vi "Elevator Controller.vi"(8 "error in":errorcluster) -> ()   [LabVIEW 2018]
doc: "This VI executes continuously carrying out the current operation and responding to updates or new operations. It will often contain the timing or control code that is difficult to place directly in TeleOp. This VI generally opens all sensors and motors and isolates the rest of the robot code from knowing how the operations are carried out."
uses:
  Elevator Setpoints.ctl
  Elevator Operations.ctl
  <vilib>/Rock Robotics/WPI/ThirdParty/Phoenix-LabVIEW/Motor Controller/Controls/CTRE_Phoenix_MotorControl_NeutralMode.ctl
  <vilib>/Rock Robotics/WPI/ThirdParty/Phoenix-LabVIEW/Motor Controller/Controls/CTRE_Phoenix_MotorControl_ControlMode.ctl
  <vilib>/Rock Robotics/WPI/ThirdParty/Phoenix-LabVIEW/Motor Controller/Controls/CTRE_Phoenix_MotorControl_FeedbackDevice.ctl
  <vilib>/Rock Robotics/SystemInterfaces/DIO/FPGA_DIOChannel.ctl
  <vilib>/Rock Robotics/WPI/ThirdParty/Phoenix-LabVIEW/Motor Controller/Get/CTRE_Phoenix_MotorController_GetQuadratureData.vi
  <vilib>/Rock Robotics/Network Tables/NT Write Number.vi
  <vilib>/Rock Robotics/Network Tables/NT Write Boolean.vi
panel:
  out "Current\nCmd":string
  # "Tip: It may be helpful to observe inputs and sensor values.\nYou may also want to display tuning or debugging controls."
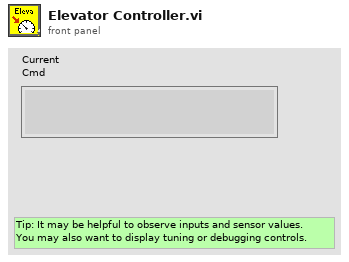
[diagram p1: front panel]
types:
  T1 = typedef "FPGA_DIOChannel.ctl" = enum8{"DIO 0", "DIO 1", "DIO 2", "DIO 3", "DIO 4", "DIO 5", "DIO 6", "DIO 7", "DIO 8", "DIO 9", "DIO MXP 0", "DIO MXP 1", "DIO MXP 2", "DIO MXP 3", "DIO MXP 4", "DIO MXP 5", "DIO MXP 6", "DIO MXP 7", "DIO MXP 8", "DIO MXP 9", "DIO MXP 10", "DIO MXP 11", "DIO MXP 12", "DIO MXP 13", "DIO MXP 14", "DIO MXP 15", "SPI Port CS1", "SPI Port CS2", "SPI Port CS3", "SPI Port MISO", "SPI Port MOSI", "Invalid"}
  T2 = typedef "CTRE_Phoenix_MotorControl_FeedbackDevice.ctl" = i8
  T3 = typedef "CTRE_Phoenix_MotorControl_ControlMode.ctl" = u16
  T4 = typedef "CTRE_Phoenix_MotorControl_NeutralMode.ctl" = enum8{"EEPROMSetting", "Override to Coast", "Override to Brake"}
  T5 = typedef "Elevator Setpoints.ctl" = cluster{"Operation":T6, "Setpoint":dbl, "Duration":dbl}
  T6 = typedef "Elevator Operations.ctl" = enum16{"Reserve", "Read Current", "Immediate", "Move Elevator", "Elevator Preset", "Elevator For Time"}
  T7 = typedef "WPI_MotorControlDeviceRef.ctl" = cluster{"DeviceStatus":errorcluster, "Type":T8, "PWM":cluster{"PWM Channel":T9, "DeadBand":T10}, "CAN":cluster{"Device Number":u8, "SetOutput VI Ref":variant, "GetOutput VI Ref":variant, "Enable VI Ref":variant, "Disable VI Ref":variant, "Data":variant}, "Invert":bool, "DIO PWM":cluster{"PWM \"Enable\" Channel":T9, "DIOChannel":T1, "PWM Rate":dbl}}
  T8 = typedef "WPI_MotorControlType.ctl" = enum16{"PWM", "CAN", "DIO PWM"}
  T9 = typedef "FPGA_DIOPWMChannel.ctl" = enum8{"PWM 0", "PWM 1", "PWM 2", "PWM 3", "PWM 4", "PWM 5", "PWM 6", "PWM 7", "PWM 8", "PWM 9", "PWM MXP 0", "PWM MXP 1", "PWM MXP 2", "PWM MXP 3", "PWM MXP 4", "PWM MXP 5", "PWM MXP 6", "PWM MXP 7", "PWM MXP 8", "PWM MXP 9", "Invalid"}
  T10 = typedef "WPI_PWMDeadband.ctl" = cluster{"Name":string, "maxPositivePwm":i32, "minPositivePwm":i32, "centerPwm":i32, "maxNegativePwm":i32, "minNegativePwm":i32, "angularRange":u16}
  T11 = typedef "Command Status Info.ctl" = cluster{"Name":string, "Status":T12, "notifier out":T13}
  T12 = typedef "Completion Status.ctl" = enum16{"Successful", "Aborted", "Incomplete"}
  T13 = typedef "Completion Notifier.ctl" = refnum<notifier>
  T14 = cluster{"Current Command":T5, "Command Timing":cluster{"Start Time (ms)":u32, "Iterations":i32}, "Command Arguments":cluster{"Command Info":T11, "Description":string, "Default Command":T5, "queue out":refnum<queue>, "Subsystem Name":string}}
  T15 = typedef "WPI_DigitalInputDevRef.ctl" = cluster{"DevStatus":errorcluster, "DIO Channel":T1}
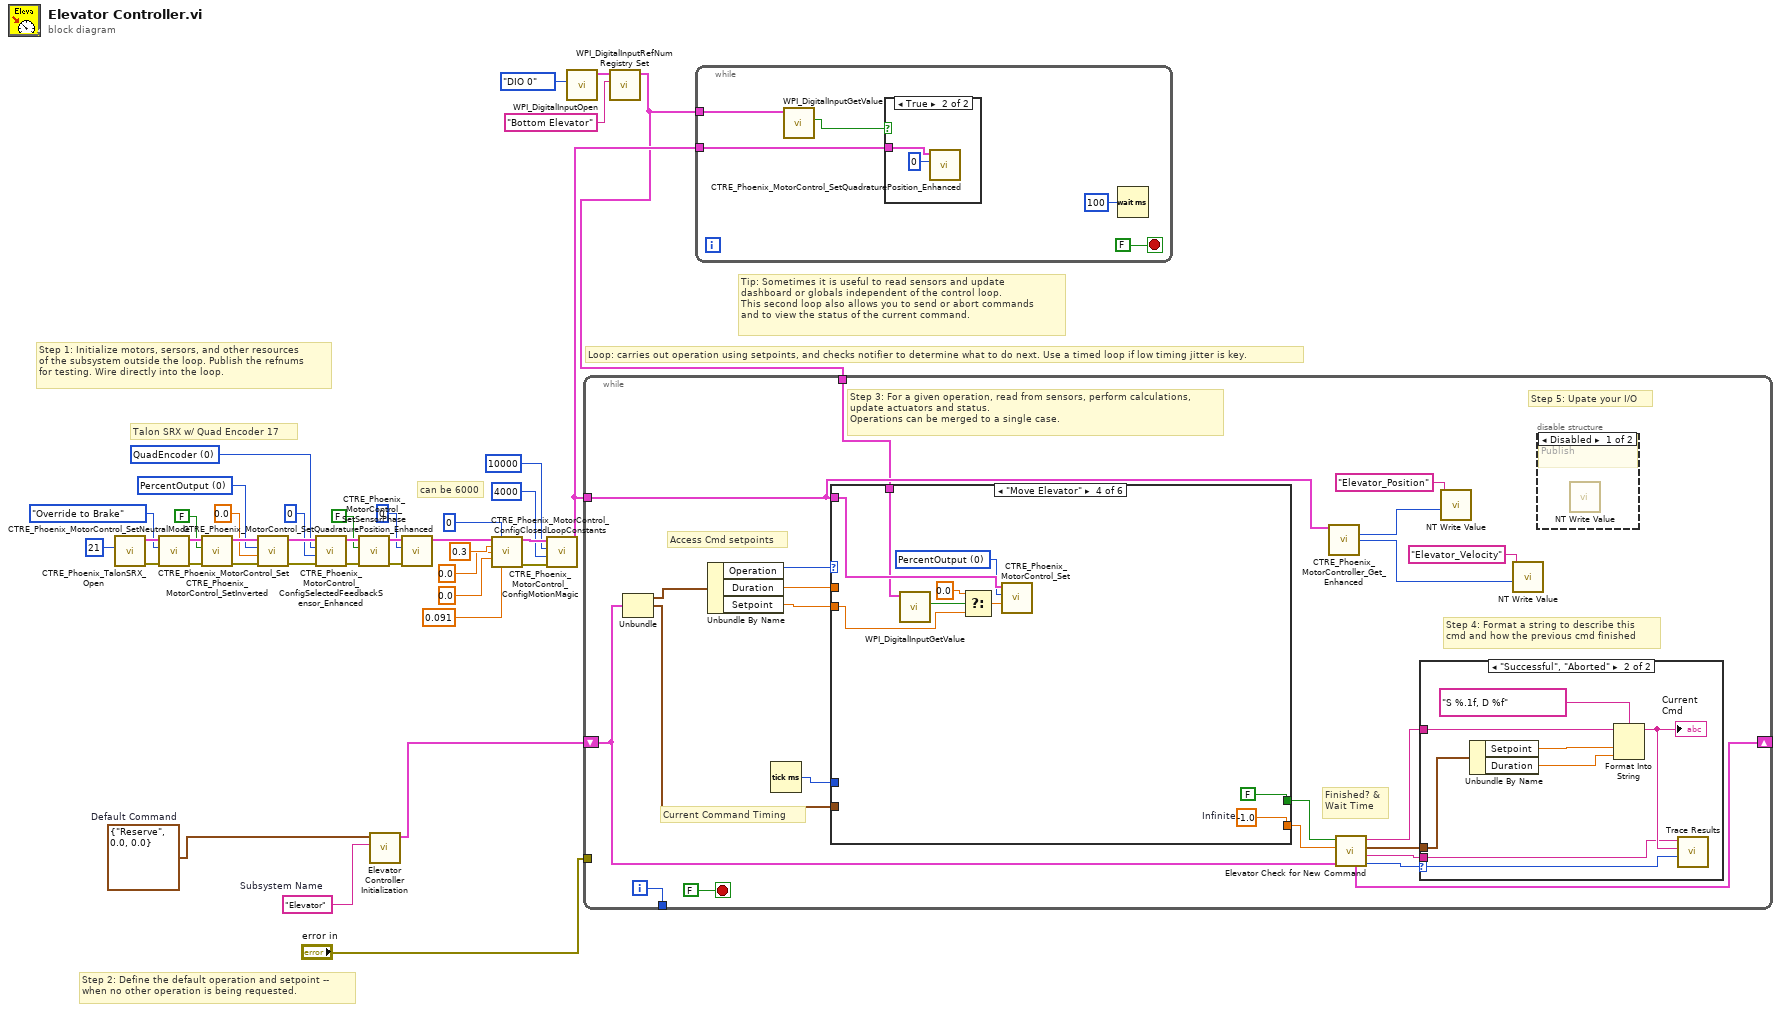
[diagram p0: block diagram]
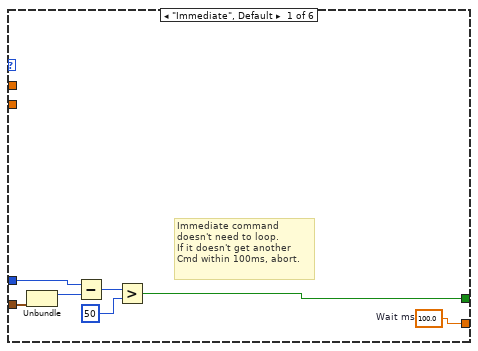
[diagram p5: hidden frame]
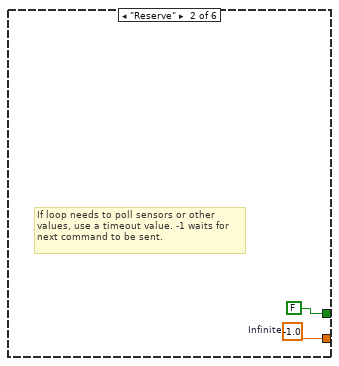
[diagram p6: hidden frame]
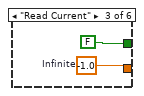
[diagram p7: hidden frame]
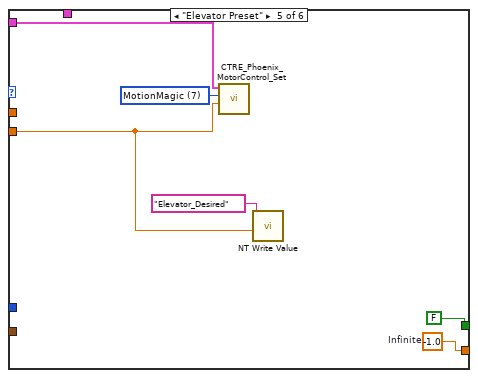
[diagram p8: hidden frame]
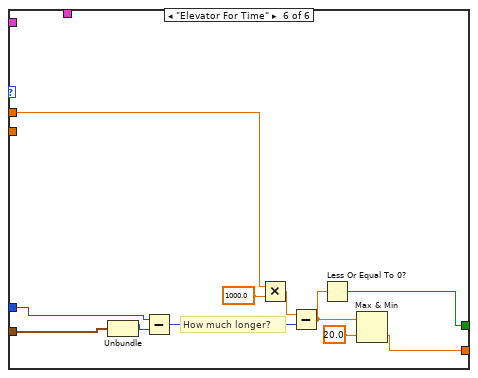
[diagram p9: hidden frame]
diagram:
  w19 = T2 0 items=["QuadEncoder"=0, "Analog"=2, "Tachometer"=4, "Pulse Width Encoded Position"=8, "Sensor Sum (S0 + S1)"=9, "Sensor Difference (D0 - D1)"=10, "Remote Source 0"=11, "Remote Source 1"=12, "Software Emulated"=15] ("Feedback Device")
  w21 = T3 0 items=["PercentOutput"=0, "Position"=1, "Velocity"=2, "Current"=3, "Follower"=5, "MotionProfile"=6, "MotionMagic"=7, "MotionProfileArc"=10, "Disabled"=15] ("Control Mode")
  w37 = T5 {"Operation"=enum."Reserve", "Setpoint"=0.0, "Duration"=0.0}  # Default Command
  w38 = "Elevator"  # Subsystem Name
  # "can be 6000"
  # "Talon SRX w/ Quad Encoder 17"
  # "Tip: Sometimes it is useful to read sensors and update\ndashboard or globals independent of the control loop.\nThis second loop also allows you to send or abort commands\nand to view the status of the current command."
  # "Step 2: Define the default operation and setpoint --\nwhen no other operation is being requested."
  # "Step 1: Initialize motors, sersors, and other resources\nof the subsystem outside the loop. Publish the refnums\nfor testing. Wire directly into the loop."
  # "Loop: carries out operation using setpoints, and checks notifier to determine what to do next. Use a timed loop if low timing jitter is key."
  n1 = call <vilib>:"CTRE_Phoenix_TalonSRX_Open.vi"("Device Number"=u8 21) -> ("error out"=w26:errorcluster, "CAN Talon SRX Ref"=w25:T7)  [unwired: 9 in]
  n2 = call <vilib>:"CTRE_Phoenix_MotorControl_SetNeutralMode.vi"("error in (no error)"=w26, "Motor Control Neutral Mode"=CTRE_Phoenix_MotorControl_NeutralMode."Override to Brake", "PhoenixMotorControlDevRef"=w25) -> ("error out"=w36:errorcluster, "PhoenixMotorControlDevRef"=w35:T7)  [unwired: 7 in]
  n3 = call <vilib>:"CTRE_Phoenix_MotorControl_SetInverted.vi"("error in (no error)"=w36, "Invert?"=FALSE, "PhoenixMotorControlDevRef"=w35) -> ("error out"=w34:errorcluster, "PhoenixMotorControlDevRef"=w33:T7)  [unwired: 7 in]
  n4 = call <vilib>:"CTRE_Phoenix_MotorControl_Set.vi"("error in (no error)"=w34, "Output"=0.0, "Control Mode"=w21, "PhoenixMotorControlDevRef"=w33) -> ("error out"=w27:errorcluster, "PhoenixMotorControlDevRef"=w32:T7)  [unwired: 6 in]
  n5 = call <vilib>:"CTRE_Phoenix_MotorControl_ConfigSelectedFeedbackSensor_Enhanced.vi"("error in (no error)"=w27, "pidLoopIdx"=0, "Feedback Device"=w19, "PhoenixMotorControlDevRef"=w32) -> ("error out"=w28:errorcluster, "PhoenixMotorControlDevRef"=w31:T7)  [unwired: 6 in]
  n6 = call <vilib>:"CTRE_Phoenix_MotorControl_SetSensorPhase.vi"("error in (no error)"=w28, "PhaseSensor"=FALSE, "PhoenixMotorControlDevRef"=w31) -> ("error out"=w29:errorcluster, "PhoenixMotorControlDevRef"=w30:T7)  [unwired: 7 in]
  n7 = call "Elevator Controller Initialization.vi"("Subsystem Name"=w38, "Default Command"=w37) -> ("Current Command"=w39:T14)  [unwired: 9 in]
  n8 = call <vilib>:"CTRE_Phoenix_MotorControl_SetQuadraturePosition_Enhanced.vi"("error in (no error)"=w29, "New Position"=0, "PhoenixMotorControlDevRef"=w30) -> ("PhoenixMotorControlDevRef"=w13:T7)  [unwired: 7 in, 1 out]
  n9 = call <vilib>:"CTRE_Phoenix_MotorControl_ConfigClosedLoopConstants.vi"("PhoenixMotorControlDevRef"=w13, "slotIdx"=0, "P"=0.3, "I"=0.0, "D"=0.0, "F"=0.091) -> ("PhoenixMotorControlDevRef"=w16:T7, "error out"=w17:errorcluster)  [unwired: 8 in]
  n10 = call <vilib>:"CTRE_Phoenix_MotorControl_ConfigMotionMagic.vi"("error in (no error)"=w17, "Acceleration"=4000, "Cruise Velocity"=10000, "PhoenixMotorControlDevRef"=w16) -> ("PhoenixMotorControlDevRef"=w5:T7)  [unwired: 6 in, 1 out]
  n11 = call <vilib>:"WPI_DigitalInputOpen.vi"("DIO Channel"=FPGA_DIOChannel."DIO 0") -> ("DigitalInputDevRef"=w3:T15)  [unwired: 9 in, 1 out]
  n12 = call <vilib>:"WPI_DigitalInputRefNum Registry Set.vi"("refnum name"="Bottom Elevator", "DigitalInputDevRef"=w3) -> ("DigitalInputDevRef"=w1:T15)  [unwired: 8 in, 1 out]
  n13 = while {
    shift-right: [w54] -> _
    shift-left: w39 -> [w47]
    tunnel: [w61] -> _
    tunnel: "error in" -> [_]
    tunnel: w5 -> [w46]
    tunnel: w1 -> [w41]
    i -> [w61]
    stop <- FALSE stop-if-true
    # "Step 5: Upate your I/O"
    # "Step 4: Format a string to describe this\ncmd and how the previous cmd finished"
    # "Current Command Timing"
    # "Access Cmd setpoints"
    # "Finished? &\nWait Time"
    # "Step 3: For a given operation, read from sensors, perform calculations,\nupdate actuators and status.\nOperations can be merged to a single case."
    n14 = Unbundle(w47) -> ("Current Command"=w60:T5, "Command Timing"=w56:cluster{"Start Time (ms)":u32, "Iterations":i32})  [unwired: 1 out]
    n15 = Unbundle By Name(w60) -> ("Operation"=w59:T6, "Duration"=w58:dbl, "Setpoint"=w55:dbl)
    n16 = Tick Count (ms)() -> (millisecond timer value=w57:u32)
    n17 = case shown="\"Move Elevator\"" w59 {
      tunnel: [w77 w79 w80 w89 w95 w99] -> w52
      tunnel: [w71 FALSE ("ignore previous (F)") FALSE ("ignore previous (F)") FALSE ("ignore previous (F)") FALSE ("ignore previous (F)") w98] -> w53
      tunnel: w56 -> [w73 _ _ _ _ w101]
      tunnel: w58 -> [_ _ _ _ _ w97]
      tunnel: w57 -> [w72 _ _ _ _ w100]
      tunnel: w55 -> [_ _ _ w85 w91 _]
      tunnel: w46 -> [_ _ _ w88 w93 _]
      tunnel: w41 -> [_ _ _ w82 _ _]
      frame "Immediate", Default {
        w77 = 100.0  # Wait ms
        # "Immediate command\ndoesn't need to loop.\nIf it doesn't get another\nCmd within 100ms, abort."
        n18 = Unbundle(w73) -> ("Start Time (ms)"=w76:u32)  [unwired: 1 out]
        n19 = Subtract(x=w72, y=w76) -> (x-y=w75:u32)
        n20 = Greater?(x=w75, y=u8 50 ("Left Motor")) -> (0:w71:bool)
      }
      frame "Reserve" {
        w79 = -1.0  # Infinite
        # "If loop needs to poll sensors or other\nvalues, use a timeout value. -1 waits for\nnext command to be sent."
      }
      frame "Read Current" {
        w80 = -1.0  # Infinite
      }
      frame "Move Elevator" {
        w87 = T3 0 items=["PercentOutput"=0, "Position"=1, "Velocity"=2, "Current"=3, "Follower"=5, "MotionProfile"=6, "MotionMagic"=7, "MotionProfileArc"=10, "Disabled"=15] ("Control Mode")
        w89 = -1.0  # Infinite
        n21 = call <vilib>:"WPI_DigitalInputGetValue.vi"("DigitalInputDevRef"=w82) -> ("Value"=w86:bool)  [unwired: 8 in, 2 out]
        n22 = Select(t=0.0, s=w86, f=w85) -> (s? t:f=w84:dbl)
        n23 = call <vilib>:"CTRE_Phoenix_MotorControl_Set.vi"("Output"=w84, "Control Mode"=w87, "PhoenixMotorControlDevRef"=w88) -> ()  [unwired: 7 in, 2 out]
      }
      frame "Elevator Preset" {
        w94 = T3 7 items=["PercentOutput"=0, "Position"=1, "Velocity"=2, "Current"=3, "Follower"=5, "MotionProfile"=6, "MotionMagic"=7, "MotionProfileArc"=10, "Disabled"=15] ("Control Mode")
        w95 = -1.0  # Infinite
        n24 = call <vilib>:"CTRE_Phoenix_MotorControl_Set.vi"("Output"=w91, "Control Mode"=w94, "PhoenixMotorControlDevRef"=w93) -> ()  [unwired: 7 in, 2 out]
        n25 = call-poly <vilib>:"NT Write Value.vi"("Numeric"=w91, "Name"="Elevator_Desired") -> ()  [unwired: 9 in, 1 out]
      }
      frame "Elevator For Time" {
        # "How much longer?"
        n26 = Unbundle(w101) -> ("Start Time (ms)"=w105:u32)  [unwired: 1 out]
        n27 = Subtract(x=w100, y=w105) -> (x-y=w107:u32)
        n28 = Multiply(x=w97, y=1000.0) -> (x*y=w102:dbl)
        n29 = Subtract(x=w102, y=w107) -> (x-y=w104:dbl)
        n30 = Less Or Equal To 0?(x=w104) -> (x <= 0?=w98:bool)
        n31 = Max & Min(x=w104, y=20.0) -> (min(x,y)=w99:dbl)  [unwired: 1 out]
      }
    }
    n32 = call-poly <vilib>:"CTRE_Phoenix_MotorController_Get_Enhanced.vi"("PhoenixMotorControlDevRef"=w46) -> ("Quadrature Position"=w45:i32, "Quadrature Velocity"=w42:i32)  [unwired: 11 in, 2 out]
    n33 = call "Elevator Check for New Command.vi"("Current Command"=w47, "Wait time (ms)"=w52, "Finished?"=w53) -> ("Completion"=w48:T12, "Subsystem Name"=w49:string, "Current Command"=w50:T5, "Initial Trace String"=w51:string, "NextCommand"=w54:T14)  [unwired: 4 in]
    n34 = case shown="\"Successful\", \"Aborted\"" w48 {
      selector: w48 -> [_ w70]
      tunnel: w51 -> [_ w66]
      tunnel: w50 -> [_ w67]
      tunnel: w49 -> [_ w63]
      frame "Incomplete", Default {
        # "Continuing current command"
      }
      frame "Successful", "Aborted" {
        # "Report and setup for next command"
        n35 = Unbundle By Name(w67) -> ("Setpoint"=w69:dbl, "Duration"=w64:dbl)
        n36 = Format Into String(format string="S %.1f, D %f", initial string=w66, w69, w64) -> (resulting string=w65:string)  [unwired: 1 in, 1 out]
        "Current\nCmd" <- w65
        n37 = call <vilib>:"Trace Results.vi"("Status of previous command"=w70, "Description"=w65, "Subsystem"=w63) -> ()  [unwired: 9 in]
      }
    }
    n38 = call-poly <vilib>:"NT Write Value.vi"("Numeric"=w45, "Name"="Elevator_Position") -> ()  [unwired: 9 in, 1 out]
    n39 = call-poly <vilib>:"NT Write Value.vi"("Numeric"=w42, "Name"="Elevator_Velocity") -> ()  [unwired: 9 in, 1 out]
    n40 = disable-structure shown="Disabled" {
      frame Disabled {
        # "Publish"
        n41 = call-poly <vilib>:"NT Write Value.vi"() -> ()  [unwired: 11 in, 1 out]
      }
      frame Enabled {
      }
    }
  }
  n42 = while {
    tunnel: w5 -> [w110]
    tunnel: w1 -> [w108]
    stop <- FALSE stop-if-true
    n43 = call <vilib>:"WPI_DigitalInputGetValue.vi"("DigitalInputDevRef"=w108) -> ("Value"=w109:bool)  [unwired: 8 in, 2 out]
    n44 = case shown="True" w109 {
      tunnel: w110 -> [_ w113]
      frame False {
      }
      frame True {
        n45 = call <vilib>:"CTRE_Phoenix_MotorControl_SetQuadraturePosition_Enhanced.vi"("New Position"=0, "PhoenixMotorControlDevRef"=w113) -> ()  [unwired: 8 in, 2 out]
      }
    }
    n46 = Wait (ms)(milliseconds to wait=u32 100) -> ()  [unwired: 1 out]
  }
